vi "Simulation gaussienne.vi"() -> ()   [LabVIEW 2026]
panel:
  in  "SigmaY":dbl=20.0 format="%#_13g"
  in  "sigma X":dbl=20.0 format="%#_13g"
  in  "mY":i32(slide) scale=0.0..200.0
  in  "stop":bool
  in  "mX":i32(slide) scale=0.0..250.0
  out "Tableau":dbl[][](array[numeric])
  out "Graphe d'intensité gaussienne":dbl[][](graph)
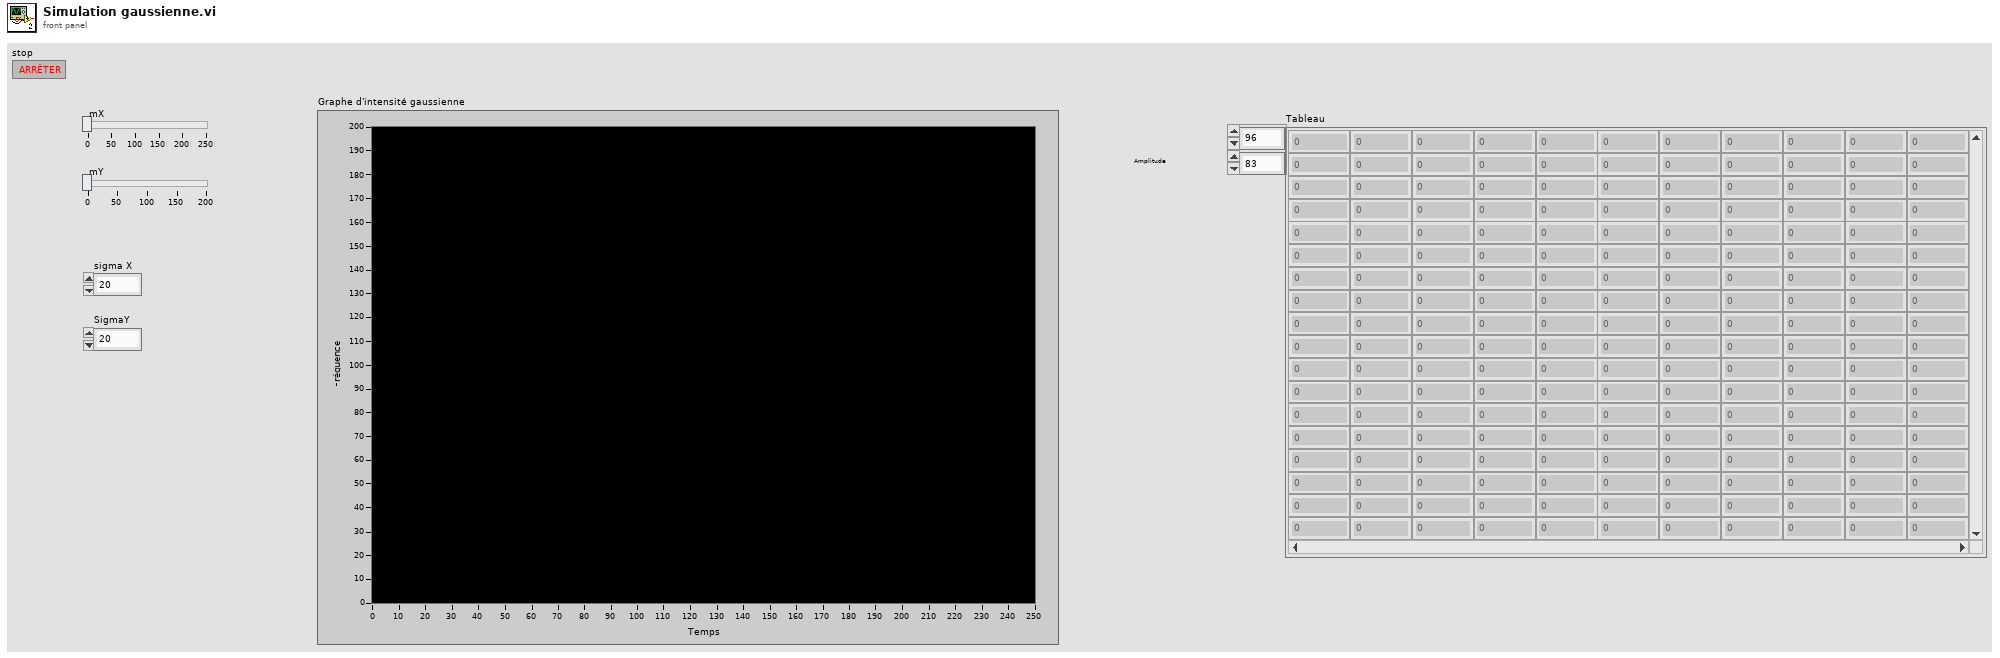
[diagram p1: front panel]
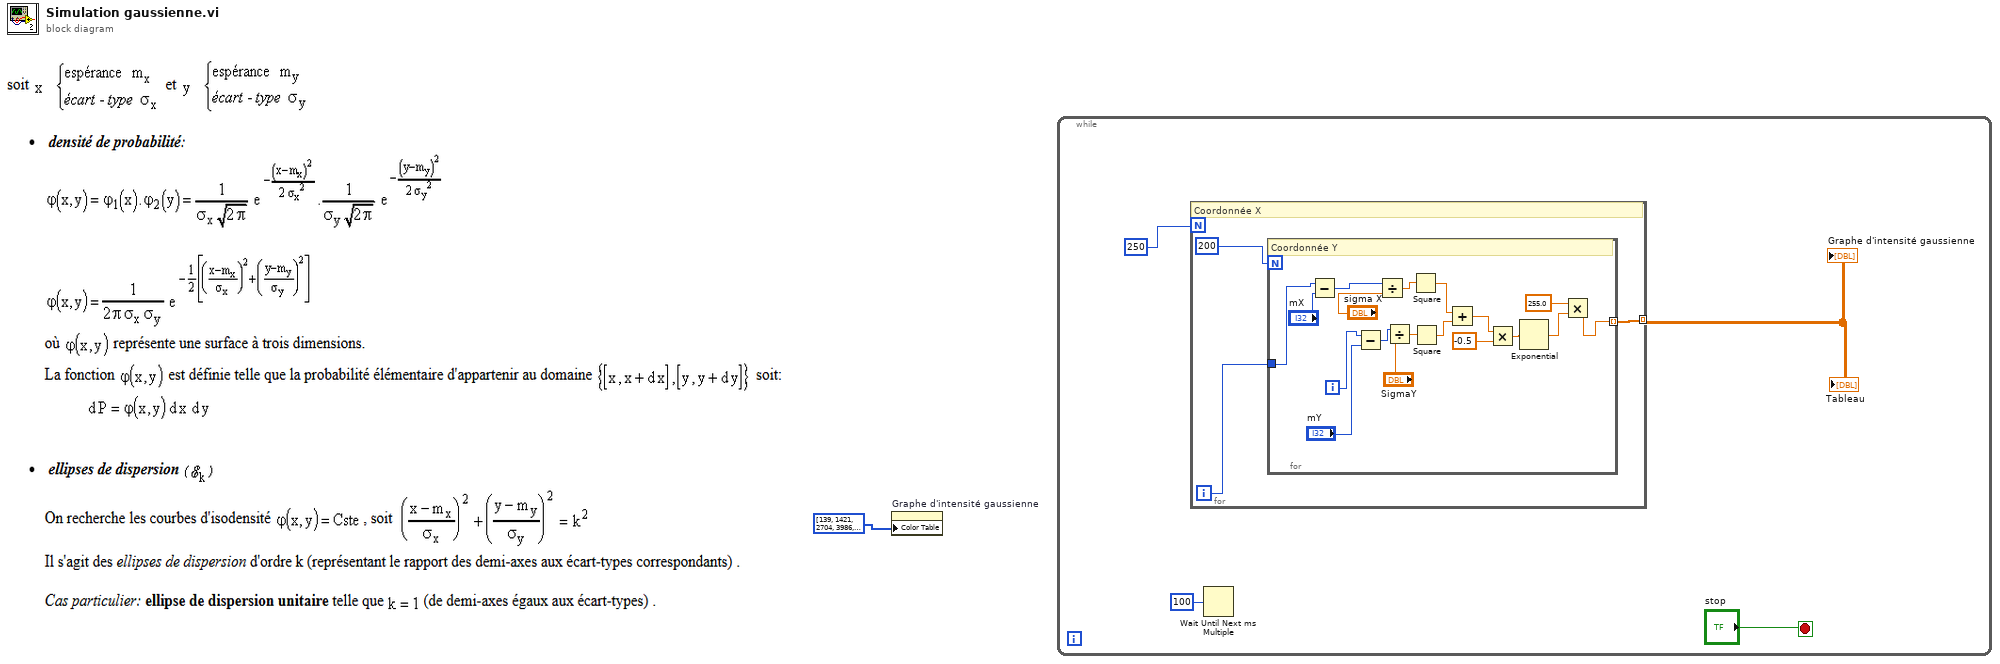
[diagram p0: block diagram]
diagram:
  n1 = property on="Graphe d'intensité gaussienne" class="GraphInt (strict)"("Color Table"=u32[] [139, 1421, 2704, 3986, 5268, 6550, 7833, 9115, 10397, 11679, 12962, 14244, 15526, 16809, 18091, 19373, 20655, 21938, 23220, 24502, 25784, 27067, 28349, 29631, 30914, 32196, 33478, 34760, 36043, 37325, 38607, 39890, 41172, 42454, 43736, 45019, 46301, 47583, 48865, 50148, 51430, 52712, 53995, 55277, 56559, 57841, 59124, 60406, 61688, 62970, 64253, 65535, 65530, 65525, 65520, 65515, 65510, 65505, 65500, 65495, 65490, 65485, 65480, 65475, 65470, 65465, 65460, 65455, 65450, 65445, 65440, 65435, 65430, 65425, 65420, 65415, 65410, 65405, 65400, 65395, 65390, 65385, 65380, 65375, 65370, 65365, 65360, 65355, 65350, 65345, 65340, 65335, 65330, 65325, 65320, 65315, 65310, 65305, 65300, 65295, 65290, 65285, 65280, 392960, 720640, 1048320, 1376000, 1703680, 2031360, 2359040, 2686720, 3014400, 3342080, 3669760, 3997440, 4325120, 4652800, 4980480, 5308160, 5635840, 5963520, 6291200, 6618880, 6946560, 7274240, 7601920, 7929600, 8257280, 8584960, 8912640, 9240320, 9568000, 9895680, 10223360, 10551040, 10878720, 11206400, 11534080, 11861760, 12189440, 12517120, 12844800, 13172480, 13500160, 13827840, 14155520, 14483200, 14810880, 15138560, 15466240, 15793920, 16121600, 16449280, 16776960, 16775680, 16774400, 16773120, 16771840, 16770560, 16769280, 16768000, 16766720, 16765440, 16764160, 16762880, 16761600, 16760320, 16759040, 16757760, 16756480, 16755200, 16753920, 16752640, 16751360, 16750080, 16748800, 16747520, 16746240, 16744960, 16743680, 16742400, 16741120, 16739840, 16738560, 16737280, 16736000, 16734720, 16733440, 16732160, 16730880, 16729600, 16728320, 16727040, 16725760, 16724480, 16723200, 16721920, 16720640, 16719360, 16718080, 16716800, 16715520, 16714240, 16712960, 16711680, 16712965, 16714250, 16715535, 16716820, 16718105, 16719390, 16720675, 16721960, 16723245, 16724530, 16725815, 16727100, 16728385, 16729670, 16730955, 16732240, 16733525, 16734810, 16736095, 16737380, 16738665, 16739950, 16741235, 16742520, 16743805, 16745090, 16746375, 16747660, 16748945, 16750230, 16751515, 16752800, 16754085, 16755370, 16756655, 16757940, 16759225, 16760510, 16761795, 16763080, 16764365, 16765650, 16766935, 16768220, 16769505, 16770790, 16772075, 16773360, 16774645, 16775930, 16777215] ("Tableau")) -> ()  [unwired: 2 in, 2 out]
  n2 = while {
    stop <- "stop" stop-if-true
    n3 = for {
      N: 250 -> [_]
      tunnel: [w6] -> w4 mode=indexing
      i -> [w7]
      # "Coordonnée X"
      n4 = for {
        N: 200 -> [_]
        tunnel: w7 -> [w16]
        tunnel: [w10] -> w6 mode=indexing
        i -> [w13]
        # "Coordonnée Y"
        n5 = Subtract(x=w16, y="mX") -> (x-y=w15:i32)
        n6 = Subtract(x=w13, y="mY") -> (x-y=w12:i32)
        n7 = Divide(x=w15, y="sigma X") -> (x/y=w23:dbl)
        n8 = Divide(x=w12, y="SigmaY") -> (x/y=w25:dbl)
        n9 = Square(x=w23) -> (x^2=w22:dbl)
        n10 = Square(x=w25) -> (x^2=w21:dbl)
        n11 = Add(x=w22, y=w21) -> (x+y=w20:dbl)
        n12 = Multiply(x=w20, y=-0.5) -> (x*y=w18:dbl)
        n13 = Exponential(1:w18) -> (0:w17:dbl)
        n14 = Multiply(x=255.0, y=w17) -> (x*y=w10:dbl)
      }
    }
    "Graphe d'intensité gaussienne" <- w4
    "Tableau" <- w4
    n15 = Wait Until Next ms Multiple(millisecond multiple=u32 100 ("n millisecondes")) -> ()  [unwired: 1 out]
  }
